vi "svfa_Convert to One-Sided Cross Spectrum.vi"(0 "two-sided cross spectrum":cdb[](array[numeric]) format="%.2f") -> (1 "one-sided cross spectrum":cdb[](array[numeric]) format="%.2f", 2 "block size":dbl format="%.2f")   [LabVIEW 2017]
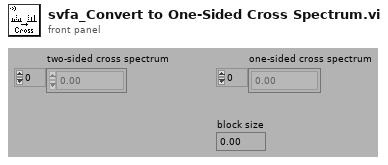
[diagram p1: front panel]
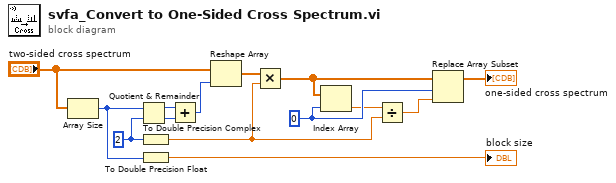
[diagram p0: block diagram]
diagram:
  w5 = 2 ("y")
  w14 = 0
  n1 = Array Size(array="two-sided cross spectrum") -> (size(s)=w9:i32)
  n2 = Quotient & Remainder(x=w9, y=w5) -> (x-y*floor(x/y)=w13:i32, floor(x/y)=w12:i32)
  n3 = To Double Precision Complex(1:w5) -> (0:w3:cdb)
  n4 = To Double Precision Float(number=w9) -> (double precision float=→"block size":dbl)
  n5 = Add(x=w13, y=w12) -> (x+y=w11:i32)
  n6 = Reshape Array("two-sided cross spectrum", w11) -> (w8:cdb[])
  n7 = Multiply(x=w8, y=w3) -> (x*y=w4:cdb[])
  n8 = Index Array(array=w4, index=w14) -> (element=w2:cdb)
  n9 = Divide(x=w2, y=w3) -> (x/y=w1:cdb)
  n10 = Replace Array Subset(array=w4, new element=w1, index=w14) -> (→"one-sided cross spectrum":cdb[])
